vi "DSF.Engine.Memory.Cache.Transfer.Get VS Channels Pointer.vi"(11 "Transfer Cache in":refnum<class "DSF.Engine.Memory.Cache.Transfer.lvclass">) -> (2 "VS Channels Pointer":refnum<class "DSF.Engine.Pointer.VS Channels.lvclass">, 3 "Transfer Cache out":refnum<class "DSF.Engine.Memory.Cache.Transfer.lvclass">)   [LabVIEW 2017, in "DSF.Engine.lvlib" / "DSF.Engine.Memory.Cache.Transfer.lvclass"]
uses:
  DSF.Engine.Memory.Cache.Transfer.lvclass
  Pointer/DSF.Engine.Pointer.VS Channels.lvclass
  DSF.Engine.Memory.Cache.Transfer.lvclass/DSF.Engine.Memory.Cache.Transfer.ctl
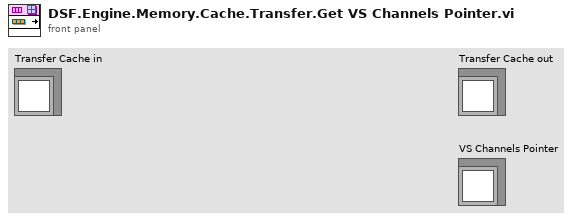
[diagram p1: front panel]
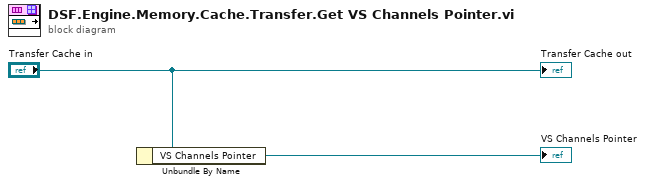
[diagram p0: block diagram]
diagram:
  n1 = Unbundle By Name("Transfer Cache in") -> ("VS Channels Pointer"=→"VS Channels Pointer":refnum<class "DSF.Engine.Pointer.VS Channels.lvclass">)
  "Transfer Cache out" <- "Transfer Cache in"
